vi "ICMP-Create.vi"(2 "Payload":u8[](array[numeric])=[97, 98, 99, 100, 101, 102, 103, 104, 105, 106, 107, 108, 109, 110, 111, 112, 113, 114, 115, 116, 117, 118, 119, 97, 98, 99, 100, 101, 102, 103, 104, 105] format="%2x", 3 "Header":T1={"Type of Message"=8, "Code"=0, "Checksum"=19779, "Quench"=65560} {"Checksum" format="%04x"}) -> (0 "ICMP Message":u8[](array[numeric])=[8, 0, 77, 67, 0, 1, 0, 24, 97, 98, 99, 100, 101, 102, 103, 104, 105, 106, 107, 108, 109, 110, 111, 112, 113, 114, 115, 116, 117, 118, 119, 97, 98, 99, 100, 101, 102, 103, 104, 105] format="%02x")   [LabVIEW 2018]
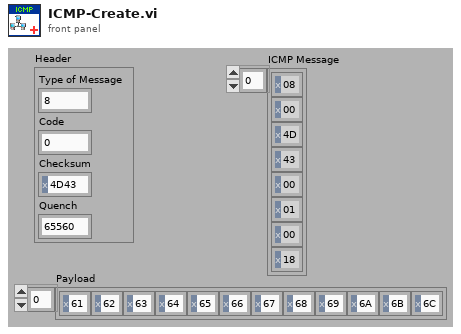
[diagram p1: front panel]
types:
  T1 = cluster{"Type of Message":u8, "Code":u8, "Checksum":u16, "Quench":u32}
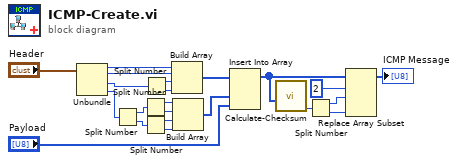
[diagram p0: block diagram]
diagram:
  n1 = Unbundle("Header") -> ("Type of Message"=w21:u8, "Code"=w20:u8, "Checksum"=w19:u16, "Quench"=w16:u32)
  n2 = Split Number(x=w16) -> (hi(x)=w14:u16, lo(x)=w15:u16)
  n3 = Split Number(x=w14) -> (hi(x)=w13:u8, lo(x)=w12:u8)
  n4 = Split Number(x=w15) -> (hi(x)=w11:u8, lo(x)=w10:u8)
  n5 = Split Number(x=w19) -> (hi(x)=w18:u8, lo(x)=w17:u8)
  n6 = Build Array(w21, w20, w18, w17) -> (w9:u8[])
  n7 = Build Array(w13, w12, w11, w10) -> (w8:u8[])
  n8 = Insert Into Array(array=w9, new element #1=w8, new element #2="Payload") -> (w6:u8[])  [unwired: 1 in]
  n9 = call "Calculate-Checksum.vi"("Array"=w6) -> ("Checksum"=w3:u16)  [unwired: 9 in, 1 out]
  n10 = Split Number(x=w3) -> (hi(x)=w2:u8, lo(x)=w1:u8)
  n11 = Replace Array Subset(array=w6, new element #1=w2, index #1=2 ("index"), new element #2=w1) -> (→"ICMP Message":u8[])  [unwired: 1 in]
